vi "ROI entry-Check Z range and adjust (single ROI).vi"(10 "AOL Z plane value":dbl, 11 "Latest Zplane_Pockels_Values file data (header removed)":dbl[](array[numeric])) -> (1 "Adjusted Z value":dbl, 2 "Z plane code":u8, 3 "Z plane Index":i32)   [LabVIEW 2017]
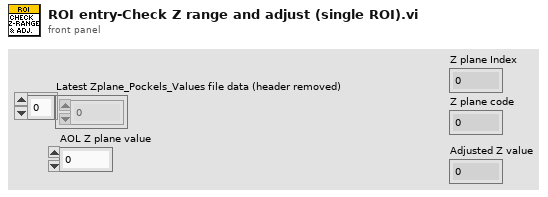
[diagram p1: front panel]
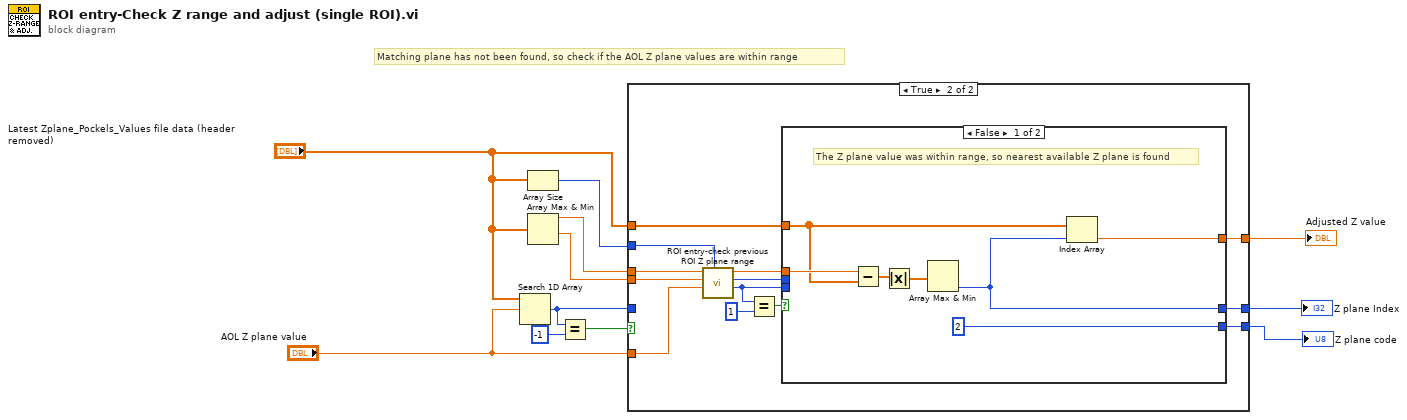
[diagram p0: block diagram]
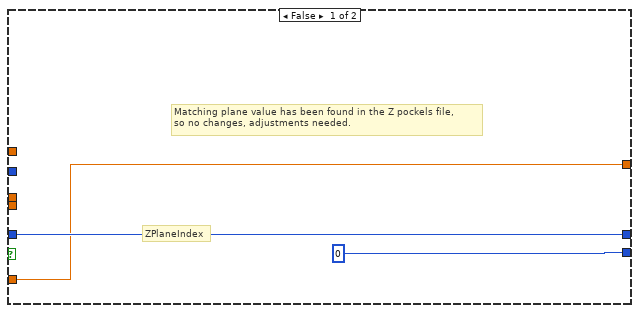
[diagram p2: hidden frame]
diagram:
  # "Matching plane has not been found, so check if the AOL Z plane values are within range"
  n1 = Search 1D Array(1D array="Latest Zplane_Pockels_Values file data (header removed)", element="AOL Z plane value") -> (index of element=w8:i32)  [unwired: 1 in]
  n2 = Array Size(array="Latest Zplane_Pockels_Values file data (header removed)") -> (size(s)=w7:i32)
  n3 = Array Max & Min(array="Latest Zplane_Pockels_Values file data (header removed)") -> (max value=w6:dbl, min value=w5:dbl)  [unwired: 2 out]
  n4 = Equal?(x=w8, y=-1) -> (x = y?=w10:bool)
  n5 = case shown="True" w10 {
    tunnel: w8 -> [w14 _]
    tunnel: w5 -> [_ w27]
    tunnel: "AOL Z plane value" -> [w12 w26]
    tunnel: w7 -> [_ w22]
    tunnel: "Latest Zplane_Pockels_Values file data (header removed)" -> [_ w19]
    tunnel: [w14 w18] -> w3
    tunnel: [u8 0 w17] -> w2
    tunnel: w6 -> [_ w16]
    tunnel: [w12 w15] -> w1
    frame False {
      # "Matching plane value has been found in the Z pockels file,\nso no changes, adjustments needed."
      # "ZPlaneIndex"
    }
    frame True {
      n6 = call "ROI entry-check previous ROI Z plane range.vi"("Z array size"=w22, "Z value"=w26, "min Z"=w27, "max Z"=w16) -> ("Code"=w20:u8, "Z plane Index"=w21:i32, "Z value"=w23:dbl)  [unwired: 4 in, 1 out]
      n7 = Equal?(x=w20, y=u8 1) -> (x = y?=w24:bool)
      n8 = case shown="False" w24 {
        tunnel: w23 -> [w32 w35]
        tunnel: w21 -> [_ w37]
        tunnel: w20 -> [_ w36]
        tunnel: w19 -> [w30 _]
        tunnel: [w29 w37] -> w18
        tunnel: [u8 2 ("y") w36] -> w17
        tunnel: [w28 w35] -> w15
        frame False {
          # "The Z plane value was within range, so nearest available Z plane is found"
          n9 = Subtract(x=w32, y=w30) -> (x-y=w34:dbl[])
          n10 = Absolute Value(x=w34) -> (abs(x)=w33:dbl[])
          n11 = Array Max & Min(array=w33) -> (min index (indices)=w29:i32)  [unwired: 3 out]
          n12 = Index Array(array=w30, index=w29) -> (element=w28:dbl)
        }
        frame True {
          # "Z plane has been coerced as it was out of range"
        }
      }
    }
  }
  "Z plane Index" <- w3
  "Z plane code" <- w2
  "Adjusted Z value" <- w1
